vi "SetModeStandard.vi"(8 "error in (no error)":errorcluster) -> (0 "error out":errorcluster)   [LabVIEW 2011]
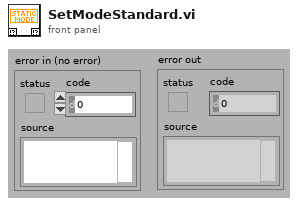
[diagram p1: front panel]
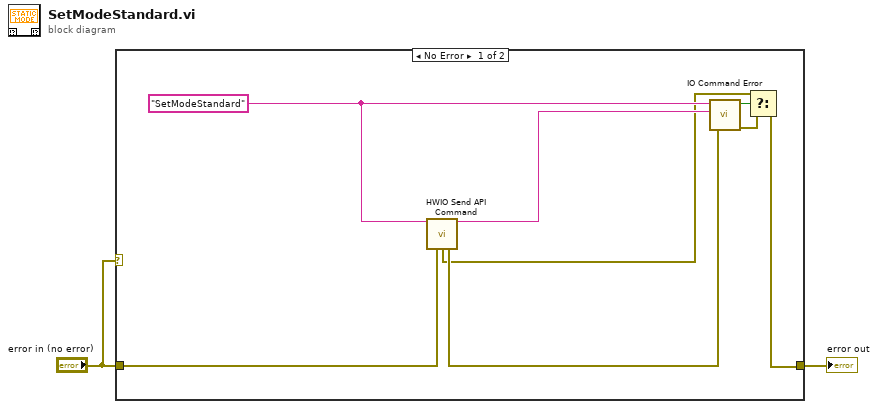
[diagram p0: block diagram]
diagram:
  n1 = case shown="No Error" "error in (no error)" {
    tunnel: "error in (no error)" -> [w10 w11]
    tunnel: [w4 w11] -> w2
    frame No Error {
      w8 = "SetModeStandard"
      n2 = call "HWIO Send API Command.vi"("Action"=w8, "error in (no error)"=w10) -> ("Action out"=w7:string, "HWError"=w3:errorcluster, "error out"=w9:errorcluster)  [unwired: 6 in, 5 out]
      n3 = call "IO Command Error.vi"("error in (no error)"=w9, "Command Returned (\"\")"=w7, "Command Sent (\"\")"=w8) -> ("error out"=w5:errorcluster, "HW ERR?"=w6:bool)  [unwired: 3 out]
      n4 = Select(t=w3, s=w6, f=w5) -> (s? t:f=w4:errorcluster)
    }
    frame Error {
    }
  }
  "error out" <- w2
